vi "Covert to Valid Folder Name.vi"(0 "Folder Name":string, 11 "error in (no error)":errorcluster) -> (4 "Valid Folder Name":string, 15 "error out":errorcluster)   [LabVIEW 2021, in "Packager Helpers.lvlib"]
uses:
  Packager Helpers.lvlib
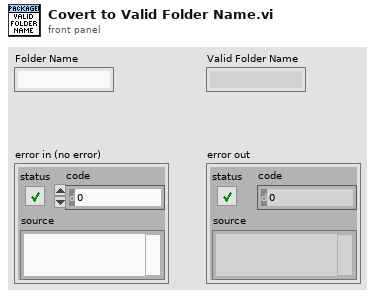
[diagram p1: front panel]
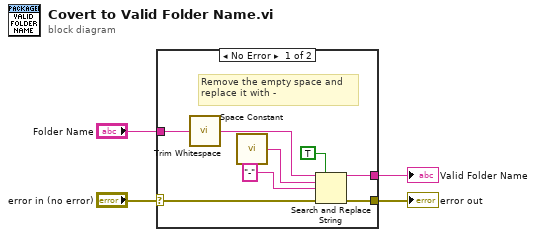
[diagram p0: block diagram]
diagram:
  n1 = case shown="No Error" "error in (no error)" {
    selector: "error in (no error)" -> [w12 w13]
    tunnel: "Folder Name" -> [w7 _]
    tunnel: [w6 _] -> w2
    tunnel: [w5 w13] -> w1
    frame No Error {
      # "Remove the empty space and\nreplace it with -"
      n2 = call <vilib>:"Trim Whitespace.vi"("string"=w7) -> ("trimmed string"=w8:string)  [unwired: 1 in]
      n3 = call <vilib>:"Space Constant.vi"() -> ("String"=w9:string)
      n4 = Search and Replace String(replace all?=TRUE ("replace all? (F)"), input string=w8, search string=w9, replace string="-" ("replace string (\"\")"), error in=w12) -> (result string=w6:string, error out=w5:errorcluster)  [unwired: 3 in, 2 out]
    }
    frame Error {
    }
  }
  "error out" <- w1
  "Valid Folder Name" <- w2
